vi "Policy Jacobian.vi"(8 "error in (no error)":errorcluster, 9 "delta":dbl=0.01, 10 "ref p":dbl[](array[numeric]), 11 "Delta Robot Kinematics in":refnum<class "Delta Robot Kinematics.lvclass">) -> (0 "error out":errorcluster, 1 "calulated":bool, 2 "Jacobian":T1, 3 "Delta Robot Kinematics out":refnum<class "Delta Robot Kinematics.lvclass">)   [LabVIEW 2013, in "Delta Robot Kinematics.lvclass"]
uses:
  Delta Robot Kinematics.lvclass
  <vilib>/Analysis/Matrix/Datatypes/RealMatrix.ctl
  <vilib>/Analysis/baseanly.llb/Real A x B.vi
  <vilib>/Analysis/7linalg.llb/Create Special Real Matrix.vi
  <vilib>/Analysis/Matrix/Numeric/Multiply/Multiply - R,RM.vi
  <vilib>/Analysis/Matrix/Numeric/Conversions/Array To Matrix - RA2.vi
  <vilib>/Analysis/Matrix/NI_Matrix.lvlib
  <vilib>/Analysis/NI_AALPro.lvlib
  <vilib>/Analysis/NI_AALBase.lvlib
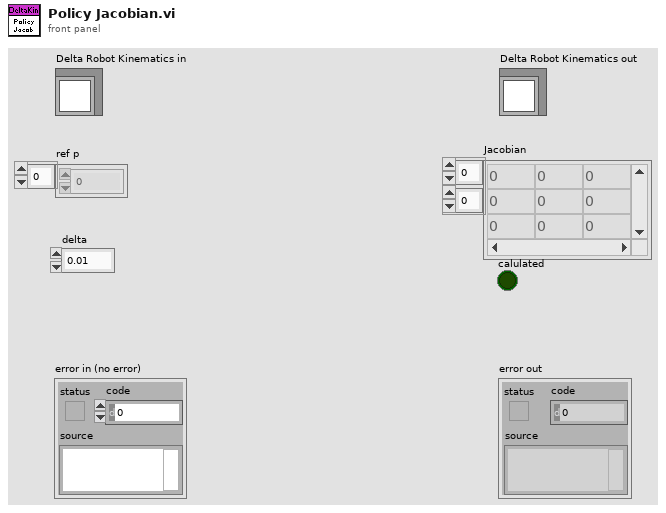
[diagram p1: front panel]
types:
  T1 = typedef "NI_Matrix.lvlib/RealMatrix.ctl" = dbl[][]
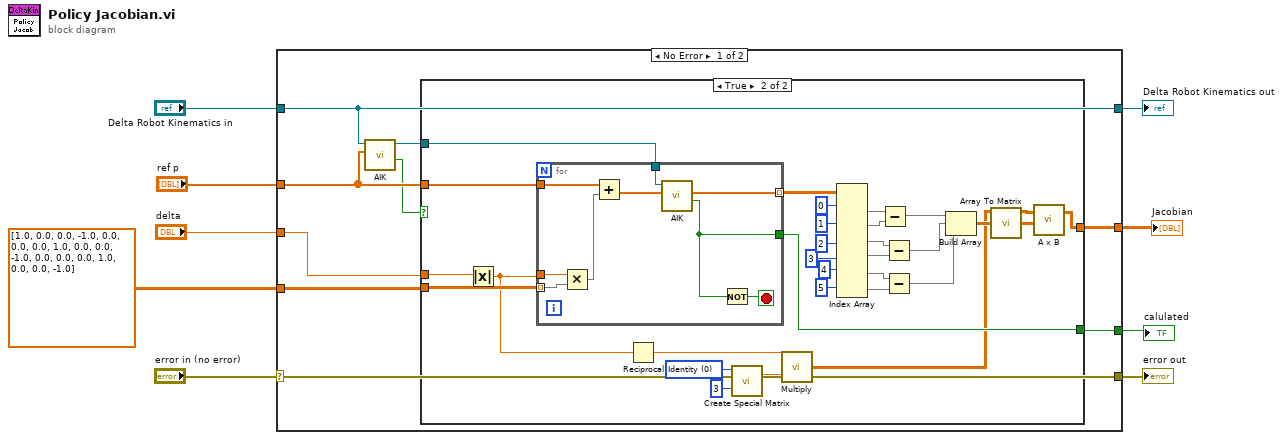
[diagram p0: block diagram]
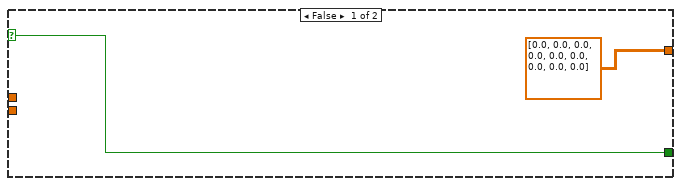
[diagram p2: hidden frame]
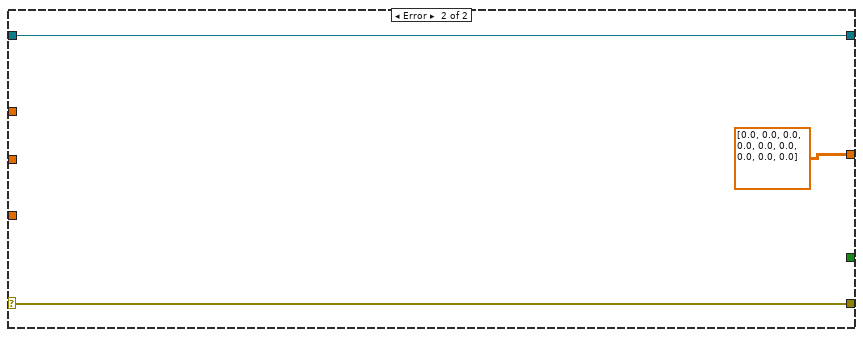
[diagram p3: hidden frame]
diagram:
  n1 = case shown="No Error" "error in (no error)" {
    selector: "error in (no error)" -> [w18 w62]
    tunnel: [w18 w62] -> w8
    tunnel: [w14 w61] -> w6
    tunnel: "Delta Robot Kinematics in" -> [w14 w61]
    tunnel: "ref p" -> [w13 _]
    tunnel: dbl[][] [[1.0, 0.0, 0.0], [-1.0, 0.0, 0.0], [0.0, 1.0, 0.0], [0.0, -1.0, 0.0], [0.0, 0.0, 1.0], [0.0, 0.0, -1.0]] -> [w17 _]
    tunnel: "delta" -> [w16 _]
    tunnel: [w15 _] -> w2
    tunnel: [w10 T1 [[0.0, 0.0, 0.0], [0.0, 0.0, 0.0], [0.0, 0.0, 0.0]] ("Real Matrix")] -> w1
    frame No Error {
      n2 = call-dynamic "AIK.vi"("p"=w13, "Delta Robot Kinematics in"=w14) -> ("exist"=w11:bool, "Delta Robot Kinematics out"=w12:refnum<class "Delta Robot Kinematics.lvclass">)  [unwired: 6 in, 2 out]
      n3 = case shown="True" w11 {
        selector: w11 -> [w20 _]
        tunnel: w17 -> [_ w50]
        tunnel: w16 -> [_ w29]
        tunnel: [w20 w49] -> w15
        tunnel: w13 -> [_ w48]
        tunnel: w12 -> [_ w47]
        tunnel: [T1 [[0.0, 0.0, 0.0], [0.0, 0.0, 0.0], [0.0, 0.0, 0.0]] ("Real Matrix") w23] -> w10
        frame False {
        }
        frame True {
          w28 = 0 items=["Identity", "Diagonal", "Toeplitz", "Vandermonde", "Companion", "Hankel", "Hadamard", "Wilkinson", "Hilbert", "Inverse Hilbert", "Rosser", "Pascal"] ("matrix type")
          n4 = Absolute Value(x=w29) -> (abs(x)=w22:dbl)
          n5 = for {
            tunnel: w50 -> [w58] mode=indexing
            tunnel: w48 -> [w59]
            tunnel: w22 -> [w57]
            tunnel: w47 -> [w55]
            tunnel: [w52] -> w49
            tunnel: [w51] -> w46 mode=indexing
            stop <- w53 stop-if-true
            n6 = Multiply(x=w57, y=w58) -> (x*y=w56:dbl[])
            n7 = Add(x=w59, y=w56) -> (x+y=w54:dbl[])
            n8 = call-dynamic "AIK.vi"("p"=w54, "Delta Robot Kinematics in"=w55) -> ("exist"=w52:bool, "joints"=w51:dbl[])  [unwired: 6 in, 2 out]
            n9 = Not(x=w52) -> (.not. x?=w53:bool)
          }
          n10 = Reciprocal(x=w22) -> (1/x=w21:dbl)
          n11 = call-poly <vilib>:"Create Special Matrix.vi"("matrix type"=w28, "matrix size"=3) -> ("Special Matrix"=w26:T1)  [unwired: 3 in, 1 out]
          n12 = call-poly <vilib>:"Multiply.vi"("Real Matrix A"=w26, "Real Scalar c"=w21) -> ("c * A"=w25:T1)
          n13 = Index Array(array=w46, index (row) #1=0 ("index (row)"), index (row) #2=1 ("index (row)"), index (row) #3=2 ("index (row)"), index (row) #4=3 ("index (row)"), index (row) #5=4 ("index (row)"), index (row) #6=5 ("index (row)")) -> (element #1=w39:dbl[], element #2=w38:dbl[], element #3=w37:dbl[], element #4=w36:dbl[], element #5=w35:dbl[], element #6=w34:dbl[])  [unwired: 6 in]
          n14 = Subtract(x=w39, y=w38) -> (x-y=w33:dbl[])
          n15 = Subtract(x=w37, y=w36) -> (x-y=w32:dbl[])
          n16 = Subtract(x=w35, y=w34) -> (x-y=w31:dbl[])
          n17 = Build Array(w33, w32, w31) -> (w30:dbl[][])
          n18 = call-poly <vilib>:"Array To Matrix.vi"("Real 2D Array"=w30) -> ("Real Matrix"=w24:T1)
          n19 = call-poly <vilib>:"A x B.vi"("B"=w24, "A"=w25) -> ("A x B"=w23:T1)  [unwired: 1 out]
        }
      }
    }
    frame Error {
    }
  }
  "error out" <- w8
  "Delta Robot Kinematics out" <- w6
  "calulated" <- w2
  "Jacobian" <- w1
